vi "IndividualSteering_main.vi"(8 "Error In":errorcluster, 10 "dt":dbl, 11 "Times In":dbl[](array[numeric]) format="%#_13g") -> (0 "Error Out":errorcluster, 2 "Servo Position":T1, 3 "Times Out":dbl[](array[numeric]))   [LabVIEW 2013]
uses:
  My Computer/Controls/Servo Position.ctl
  My Computer/Controls/Individual Steering.ctl
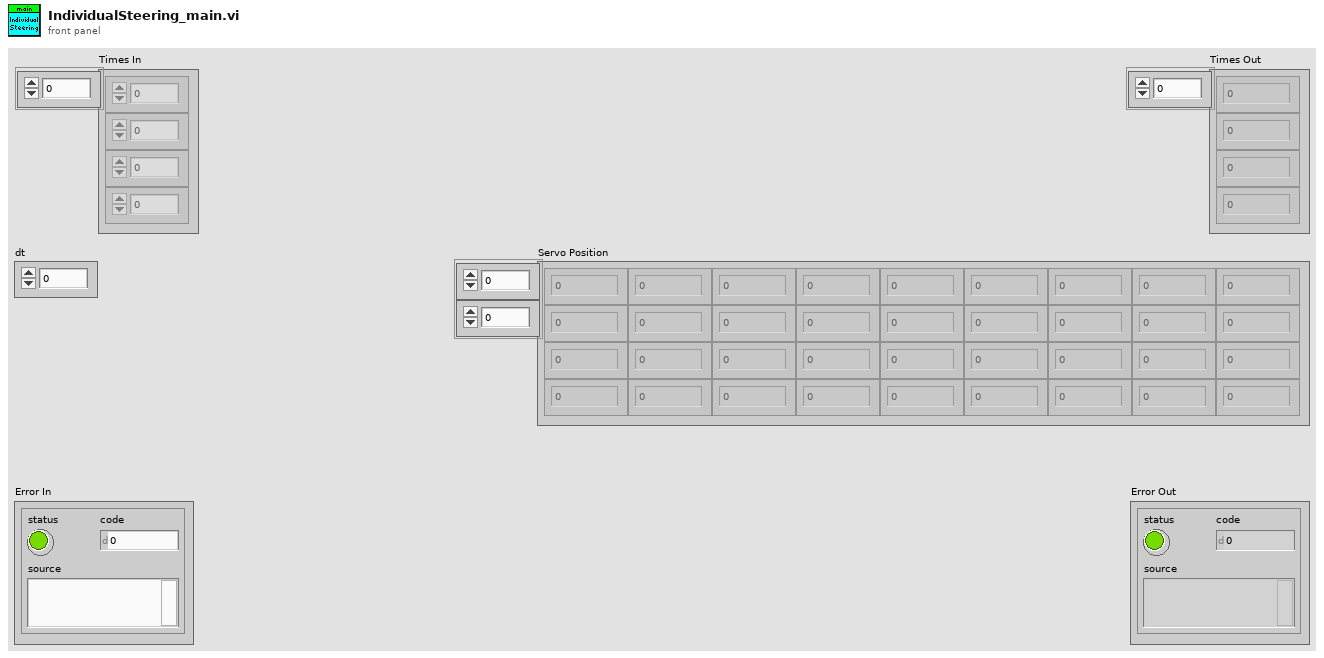
[diagram p1: front panel]
types:
  T1 = typedef "Servo Position.ctl" = dbl[][]
  T2 = typedef "Individual Steering.ctl" = cluster{"Fin Parameters":cluster{"Amplitude":dbl, "Phase Shift":dbl, "Zero Position":dbl}[], "Frequency\n& Direction":dbl, "General A, PS, ZP":cluster{"Amplitude":dbl, "Phase Shift":dbl, "Zero Position":dbl}}[]
  T3 = cluster{"Amplitude":dbl, "Phase Shift":dbl, "Zero Position":dbl}[]
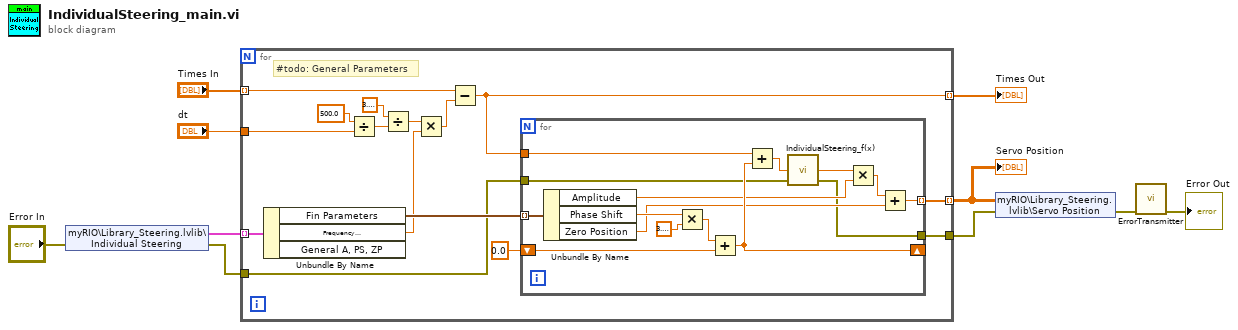
[diagram p0: block diagram]
diagram:
  n1 = shared-variable "myRIO\\Library_Steering.lvlib\\Individual Steering"(error in="Error In") -> (w4:T2, error out=w2:errorcluster)
  n2 = for {
    tunnel: w4 -> [w25] mode=indexing
    tunnel: "dt" -> [w18]
    tunnel: [w15] -> w7 mode=indexing
    tunnel: [w14] -> w6 mode=indexing
    tunnel: "Times In" -> [w13] mode=indexing
    tunnel: w2 -> [w12]
    tunnel: [w11] -> w1
    # "#todo: General Parameters"
    n3 = Unbundle By Name(w25) -> ("Fin Parameters"=w24:T3, "Frequency\n& Direction"=w17:dbl)  [unwired: 1 out]
    n4 = Divide(x=500.0, y=w18) -> (x/y=w23:dbl)
    n5 = Divide(x=3.141592653589793, y=w23) -> (x/y=w20:dbl)
    n6 = Multiply(x=w20, y=w17) -> (x*y=w21:dbl)
    n7 = Subtract(x=w13, y=w21) -> (x-y=w14:dbl)
    n8 = for {
      tunnel: w24 -> [w40] mode=indexing
      shift-right: [w35] -> _
      shift-left: 0.0 ("y") -> [w36]
      tunnel: w14 -> [w34]
      tunnel: [w30] -> w15 mode=indexing
      tunnel: w12 -> [w27]
      tunnel: [w26] -> w11
      n9 = Unbundle By Name(w40) -> ("Amplitude"=w33:dbl, "Phase Shift"=w38:dbl, "Zero Position"=w31:dbl)
      n10 = Multiply(x=w38, y=3.141592653589793) -> (x*y=w37:dbl)
      n11 = Add(x=w37, y=w36) -> (x+y=w35:dbl)
      n12 = Add(x=w34, y=w35) -> (x+y=w29:dbl)
      n13 = call "IndividualSteering_f(x).vi"("Error In"=w27, "x"=w29) -> ("Error Out"=w26:errorcluster, "y = f(x)"=w28:dbl)  [unwired: 2 in]
      n14 = Multiply(x=w28, y=w33) -> (x*y=w32:dbl)
      n15 = Add(x=w32, y=w31) -> (x+y=w30:dbl)
    }
  }
  "Servo Position" <- w7
  "Times Out" <- w6
  n16 = shared-variable "myRIO\\Library_Steering.lvlib\\Servo Position"(w7, error in=w1) -> (error out=w8:errorcluster)
  n17 = call "ErrorTransmitter.vi"("Error In"=w8) -> ("Error Out"=→"Error Out":errorcluster)  [unwired: 10 in]
